vi "Fixed-Point Configuration-part2.vi"() -> ()   [LabVIEW 2012]
uses:
  <vilib>/rvi/eio/common/nirviEmuTemplateMethod_errors.vi
  <vilib>/eio/EIONode/EIONode.xnode
panel:
  out "Result":fxp<+/-,25,5>
  out "Simulated AI0":fxp<+/-,24,4>
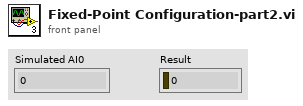
[diagram p1: front panel]
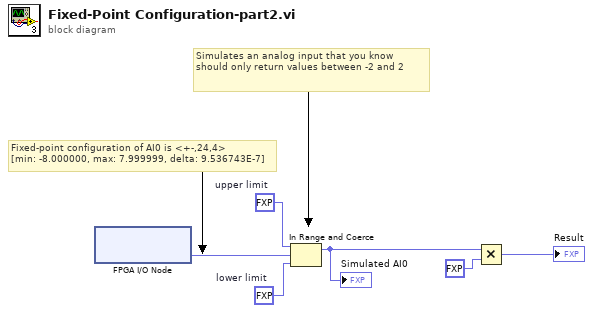
[diagram p0: block diagram]
diagram:
  w4 = fxp<+/-,24,4> -7.0  # lower limit
  w5 = fxp<+/-,24,4> 7.0  # upper limit
  # "Simulates an analog input that you know should only return values between -2 and 2"
  # "Fixed-point configuration of AI0 is <+-,24,4>\n[min: -8.000000, max: 7.999999, delta: 9.536743E-7]"
  n1 = xnode "FPGA I/O Node"() -> ("Mod2/AI0"=w6:fxp<+/-,24,4>)  [unwired: 1 in, 1 out]
  n2 = In Range and Coerce(upper limit=w5, x=w6, lower limit=w4) -> (coerced(x)=w3:fxp<+/-,24,4>)  [unwired: 1 out]
  "Simulated AI0" <- w3
  n3 = Multiply(x=w3, y=fxp<+,3,3> 5.0) -> (x*y=→"Result":fxp<+/-,25,5>)
